vi "Ohaus Scout Pro (com2).vi"(4 "State":i16, 5 "Time":dbl format="%.2f", 6 "Sensor Values":dbl[](array[numeric]), 7 "Set Points":dbl[](array[numeric])) -> (0 "required data":T2, 3 "output value":dbl)   [LabVIEW 2015]
panel:
  in  "Units (0: Gram)":u16(ring) items=["Gram (g)", "Ounce (oz)", "Troy Ounce (oz t)", "Pennyweight (dwt)", "Parts Counting (PC)", "Pound (lb)", "Newton (N)", "Kilogram (kg)", "lb or oz on some models", "Percent (%)"]
  in  "error in (no error)":errorcluster
  in  "Serial Configuration":T1={"Baud Rate (2400)"=2400, "Flow Control (2: RTS/CTS)"=2, "Parity (0: None)"=0, "Data Bits (7)"=7} {"Data Bits (7)" items=["7"=7, "8"=8]; "Parity (0: None)" items=["None", "Odd", "Even"]; "Flow Control (2: RTS/CTS)" items=["None", "XON/XOFF", "RTS/CTS"]; "Baud Rate (2400)" items=["600"=600, "1200"=1200, "2400"=2400, "4800"=4800, "9600"=9600, "19200"=19200]}
  out "VISA resource name out":refnum<visa-resource-name>
  # "Enter the correct information for this control code in the required data structure below. Then make the current value default by right clicking on the border of the data structure. Select \"data operations\" and then select \"make current value default\". These values will be displayed by process controller."
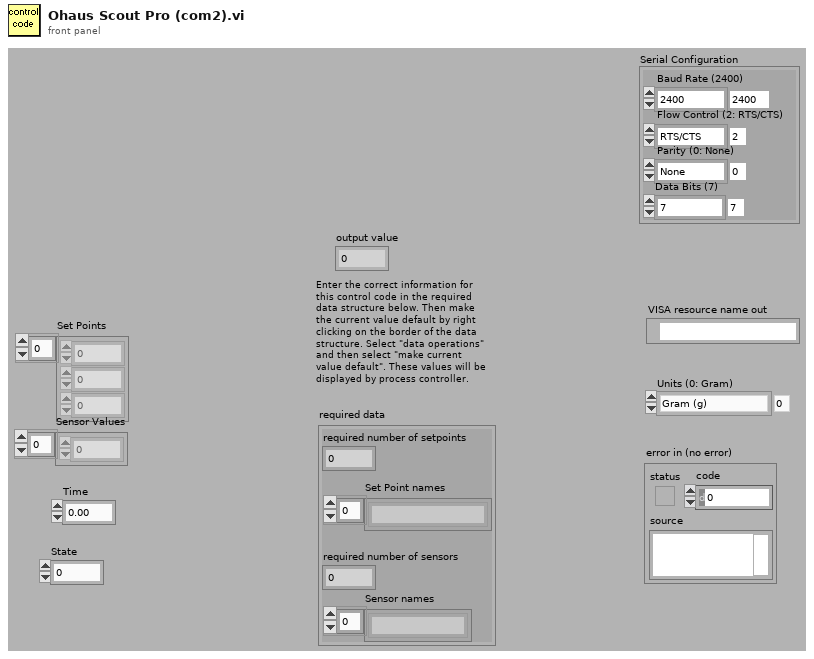
[diagram p1: front panel]
types:
  T1 = cluster{"Baud Rate (2400)":u32, "Flow Control (2: RTS/CTS)":u16, "Parity (0: None)":u16, "Data Bits (7)":u16}
  T2 = cluster{"Set Point names":string[], "required number of setpoints":u8, "required number of sensors":u8, "Sensor names":string[]}
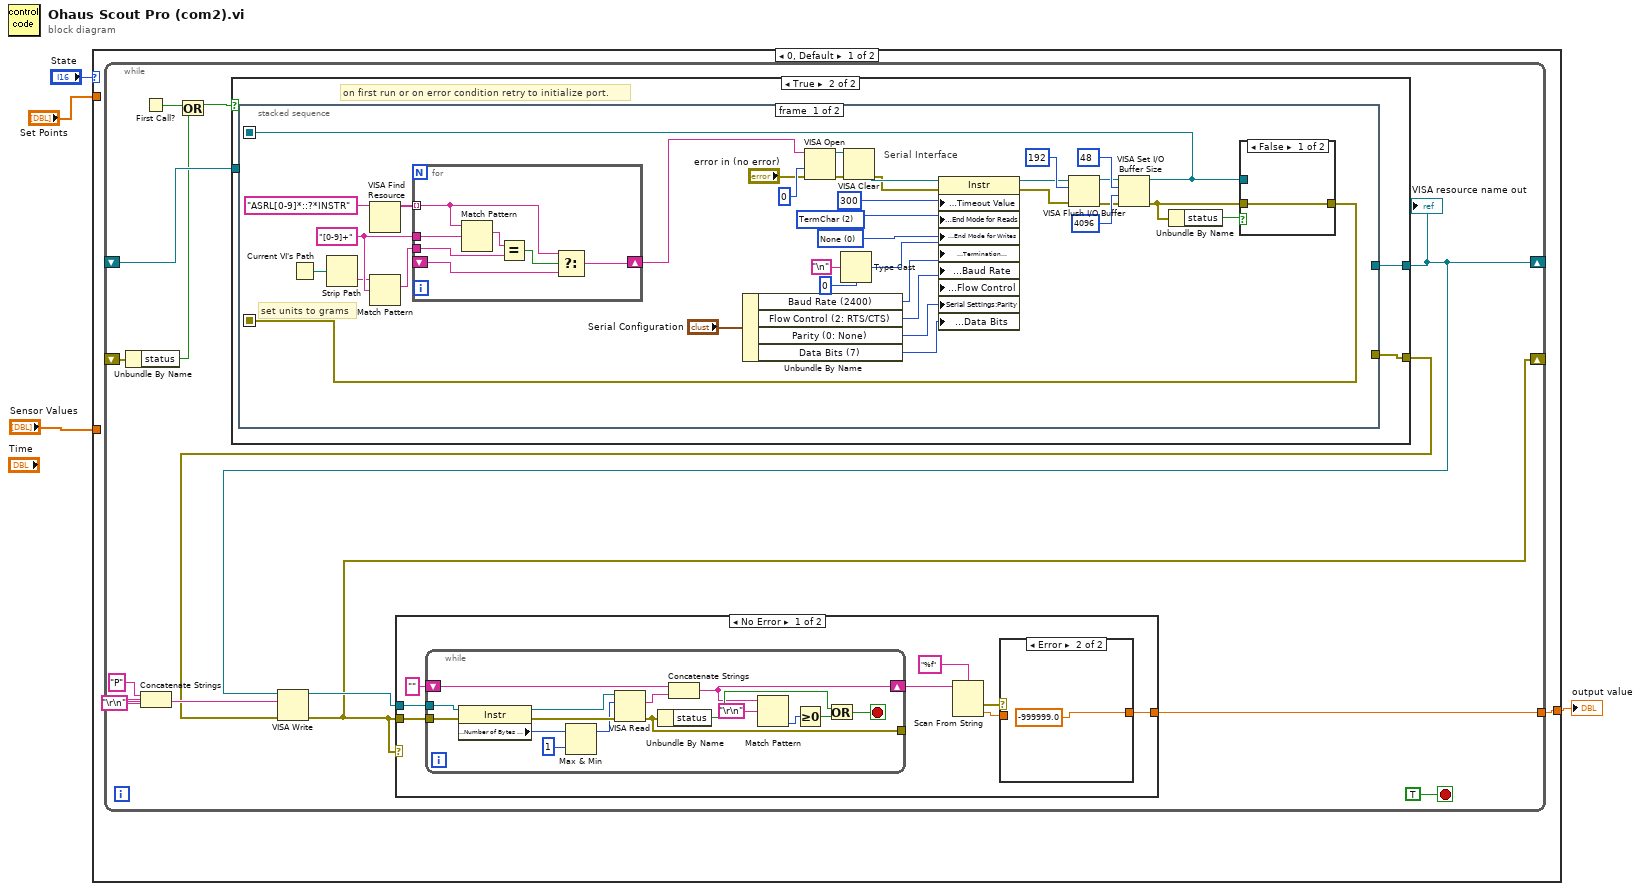
[diagram p0: block diagram]
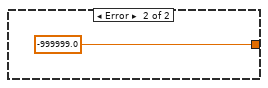
[diagram p3: hidden frame]
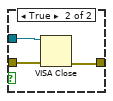
[diagram p5: hidden frame]
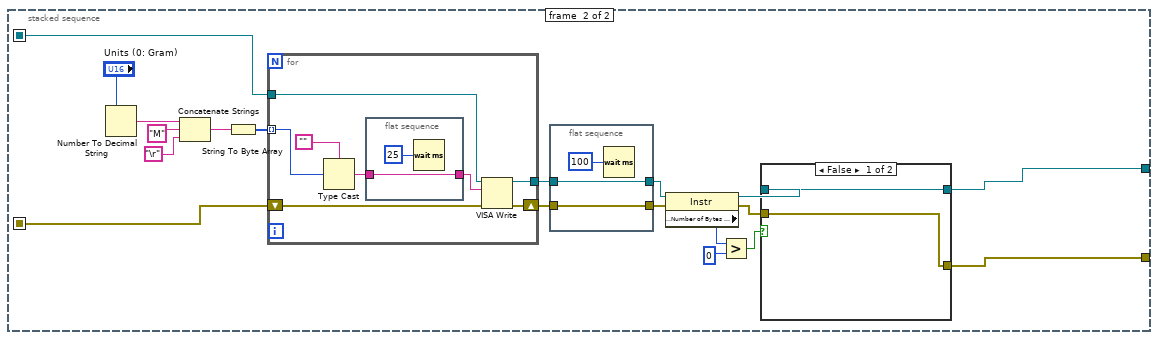
[diagram p6: hidden frame]
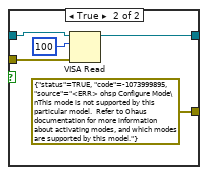
[diagram p7: hidden frame]
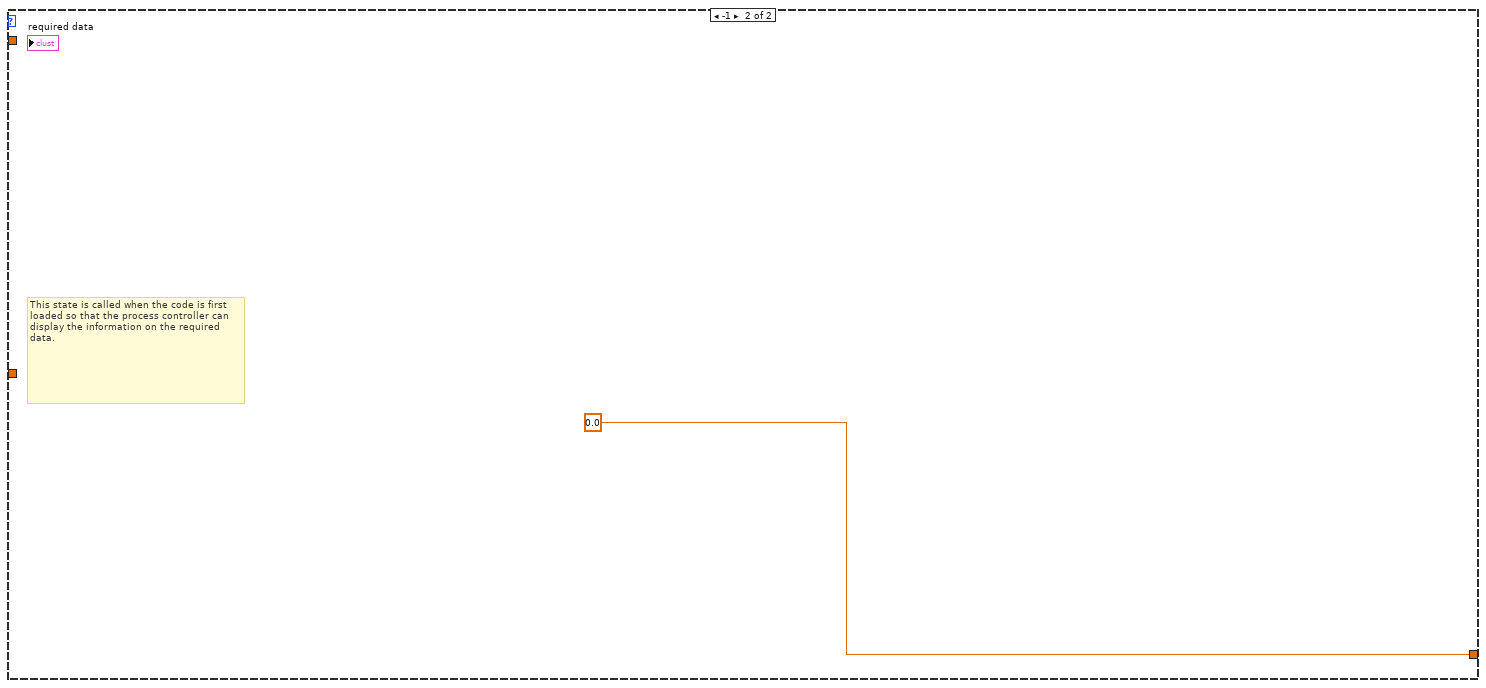
[diagram p8: hidden frame]
diagram:
  n1 = case shown="0, Default" "State" {
    tunnel: [w5 0.0 ("fraction on")] -> w3
    tunnel: "Set Points" -> [_ _]
    tunnel: "Sensor Values" -> [_ _]
    frame 0, Default {
      n2 = while {
        tunnel: [w19] -> w5
        shift-right: [w12] -> _
        shift-left: _ -> [w13]
        shift-right: [w6] -> _
        shift-left: _ -> [w9]
        stop <- TRUE stop-if-true
        n3 = Unbundle By Name(w9) -> ("status"=w7:bool)
        n4 = First Call?() -> (First Call?: T/F=w17:bool)
        n5 = Concatenate Strings("P", "\r\n") -> (w14:string)
        n6 = Or(x=w17, y=w7) -> (x .or. y?=w8:bool)
        n7 = case shown="True" w8 {
          tunnel: [_ w48] -> w10
          tunnel: [w47 w49] -> w12
          tunnel: w13 -> [w47 _]
          frame False {
          }
          frame True {
            # "on first run or on error condition retry to initialize port."
            n8 = stacked-sequence {
              seq-local: [w58 _] -> [_ w99]
              seq-local: [w57 _] -> [_ w98]
              tunnel: [_ w97] -> w49
              tunnel: [_ w96] -> w48
              frame #0 {
                w56 = "[0-9]+" ("regular expression")
                w83 = u16 0 items=["None", "LastBit", "TermChar", "Break"] ("Serial Settings:Serial End Mode for Writes")
                w73 = u16 2 items=["None", "LastBit", "TermChar"] ("Serial Settings:Serial End Mode for Reads")
                # "set units to grams"
                # "Serial Interface"
                n9 = Current VI's Path() -> (path=w51:path)
                n10 = Strip Path(path=w51) -> (name=w52:string)  [unwired: 1 out]
                n11 = VISA Find Resource(11:"ASRL[0-9]*::?*INSTR" ("expression (\"?*\")")) -> (3:w54:string[])  [unwired: 2 in, 2 out]
                n12 = Match Pattern(string=w52, regular expression=w56) -> (match substring=w55:string)  [unwired: 1 in, 3 out]
                n13 = for {
                  tunnel: w54 -> [w86] mode=indexing
                  tunnel: w55 -> [w90]
                  shift-right: [w87] -> w50
                  shift-left: _ -> [w88]
                  tunnel: w56 -> [w85]
                  n14 = Match Pattern(string=w86, regular expression=w85) -> (match substring=w91:string)  [unwired: 1 in, 3 out]
                  n15 = Equal?(x=w91, y=w90) -> (x = y?=w89:bool)
                  n16 = Select(t=w86, s=w89, f=w88) -> (s? t:f=w87:string)
                }
                n17 = Unbundle By Name("Serial Configuration") -> ("Baud Rate (2400)"=w76:u32, "Flow Control (2: RTS/CTS)"=w77:u16, "Parity (0: None)"=w79:u16, "Data Bits (7)"=w78:u16)
                n18 = VISA Open(access mode=u32 0, error in (no error)="error in (no error)", VISA resource name=w50) -> (VISA resource name=w61:refnum<visa-resource-name>, error out=w62:errorcluster)  [unwired: 2 in]
                n19 = Type Cast(type=u8 0, x="\n" ("Line Feed Constant")) -> (*(type *) &x=w74:u8)
                n20 = VISA Clear(VISA resource name=w61, error in (no error)=w62) -> (VISA resource name out=w82:refnum<visa-resource-name>, error out=w81:errorcluster)
                n21 = property class="Instr"(reference=w82, error in=w81, "General Settings:Timeout Value"=u32 300, "Serial Settings:End Mode for Reads"=w73, "Serial Settings:End Mode for Writes"=w83, "Message Based Settings:Termination Character"=w74, "Serial Settings:Baud Rate"=w76, "Serial Settings:Flow Control"=w77, "Serial Settings:Parity"=w79, "Serial Settings:Data Bits"=w78) -> (reference out=w67:refnum<visa-resource-name>, error out=w65:errorcluster)
                n22 = VISA Flush I/O Buffer(VISA resource name=w67, mask (16)=u16 192, error in (no error)=w65) -> (VISA resource name out=w64:refnum<visa-resource-name>, error out=w66:errorcluster)
                n23 = VISA Set I/O Buffer Size(VISA resource name=w64, mask (16)=u16 48, size (4096)=u32 4096 ("size (0)"), error in (no error)=w66) -> (VISA resource name out=w58:refnum<visa-resource-name>, error out=w84:errorcluster)
                n24 = Unbundle By Name(w84) -> ("status"=w63:bool)
                n25 = case shown="False" w63 {
                  tunnel: w58 -> [_ w95]
                  tunnel: [w92 w93] -> w57
                  tunnel: w84 -> [w92 w94]
                  frame False {
                  }
                  frame True {
                    n26 = VISA Close(VISA resource name=w95, error in (no error)=w94) -> (error out=w93:errorcluster)
                  }
                }
              }
              frame #1 {
                n27 = Number To Decimal String(number="Units (0: Gram)") -> (decimal integer string=w113:string)  [unwired: 1 in]
                n28 = Concatenate Strings(w113, "M" ("string"), "\r") -> (w109:string)
                n29 = String To Byte Array(string=w109) -> (unsigned byte array=w108:u8[])
                n30 = for {
                  tunnel: w108 -> [w117] mode=indexing
                  tunnel: [w122] -> w111
                  tunnel: w99 -> [w120]
                  shift-right: [w121] -> w112
                  shift-left: w98 -> [w119]
                  n31 = Type Cast(type="", x=w117) -> (*(type *) &x=w116:string)
                  n32 = flat-sequence {
                    tunnel: w116 -> [w123]
                    tunnel: [w123] -> w115
                    frame #0 {
                      n33 = Wait (ms)(milliseconds to wait=u32 25) -> ()  [unwired: 1 out]
                    }
                  }
                  n34 = VISA Write(VISA resource name=w120, write buffer=w115, error in (no error)=w119) -> (VISA resource name out=w122:refnum<visa-resource-name>, error out=w121:errorcluster)  [unwired: 1 out]
                }
                n35 = flat-sequence {
                  tunnel: [w127] -> w106
                  tunnel: w112 -> [w127]
                  tunnel: [w125] -> w107
                  tunnel: w111 -> [w125]
                  frame #0 {
                    n36 = Wait (ms)(milliseconds to wait=u32 100) -> ()  [unwired: 1 out]
                  }
                }
                n37 = property class="Instr"(reference=w107, error in=w106) -> (reference out=w104:refnum<visa-resource-name>, error out=w105:errorcluster, "Serial Settings:Number of Bytes at Serial Port"=w103:u32)
                n38 = Greater?(x=w103, y=u32 0) -> (0:w102:bool)
                n39 = case shown="False" w102 {
                  tunnel: w104 -> [w129 w134]
                  tunnel: w105 -> [w128 w133]
                  tunnel: [w129 w132] -> w97
                  tunnel: [w128 errorcluster {"status"=TRUE, "code"=-1073999895, "source"="<ERR> ohsp Configure Mode\nThis mode is not supported by this particular model.  Refer to Ohaus documentation for more information about activating modes, and which modes are supported by this model."} ("error out")] -> w96
                  frame False {
                  }
                  frame True {
                    n40 = VISA Read(VISA resource name=w134, byte count=u32 100, error in (no error)=w133) -> (VISA resource name out=w132:refnum<visa-resource-name>)  [unwired: 3 out]
                  }
                }
              }
            }
          }
        }
        "VISA resource name out" <- w12
        n41 = VISA Write(VISA resource name=w12, write buffer=w14, error in (no error)=w10) -> (VISA resource name out=w18:refnum<visa-resource-name>, error out=w6:errorcluster)  [unwired: 1 out]
        n42 = case shown="No Error" w6 {
          tunnel: [w20 -999999.0] -> w19
          tunnel: w18 -> [w27 _]
          tunnel: w6 -> [w26 _]
          frame No Error {
            n43 = while {
              tunnel: w27 -> [w44]
              tunnel: w26 -> [w42]
              shift-right: [w30] -> w23
              shift-left: "" ("write buffer") -> [w45]
              tunnel: [w31] -> _
              stop <- w40 stop-if-true
              n44 = property class="Instr"(reference=w44, error in=w42) -> (reference out=w43:refnum<visa-resource-name>, error out=w41:errorcluster, "Serial Settings:Number of Bytes at Serial Port"=w33:u32)
              n45 = Max & Min(x=w33, y=u32 1) -> (max(x,y)=w34:u32)  [unwired: 1 out]
              n46 = VISA Read(VISA resource name=w43, byte count=w34, error in (no error)=w41) -> (read buffer=w38:string, error out=w31:errorcluster)  [unwired: 2 out]
              n47 = Unbundle By Name(w31) -> ("status"=w39:bool)
              n48 = Concatenate Strings(w45, w38) -> (w30:string)
              n49 = Match Pattern(string=w30, regular expression="\r\n") -> (offset past match=w36:i32)  [unwired: 1 in, 3 out]
              n50 = Greater Or Equal To 0?(x=w36) -> (x >= 0?=w35:bool)
              n51 = Or(x=w39, y=w35) -> (x .or. y?=w40:bool)
            }
            n52 = Scan From String(format string="%f", input string=w23) -> (error out=w22:errorcluster, output 1=w21:dbl)  [unwired: 3 in, 2 out]
            n53 = case shown="Error" w22 {
              tunnel: [w28 -999999.0] -> w20
              tunnel: w21 -> [w28 _]
              frame No Error {
              }
              frame Error {
              }
            }
          }
          frame Error {
          }
        }
      }
    }
    frame -1 {
      # "This state is called when the code is first loaded so that the process controller can display the information on the required data."
    }
  }
  "output value" <- w3
